vi "API String - Set Float Format String.vi"(8 "Error in":errorcluster caption="Error in (no error)", 11 "Float Format String Setting":string="%.6p") -> (0 "Error out":errorcluster, 3 "Float Format String":string)   [LabVIEW 2017, in "API String Arguments Support.lvlib"]
uses:
  API String Arguments Support.lvlib
  <userlib>/_NEVSTOP/Communicable State Machine(CSM)/Communicable State Machine.lvlib
  <userlib>/_NEVSTOP/Communicable State Machine(CSM)/_Shared/CSM Shared.lvlib
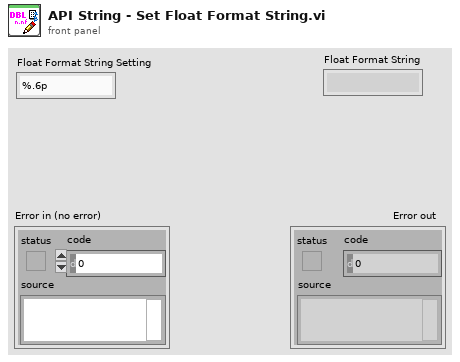
[diagram p1: front panel]
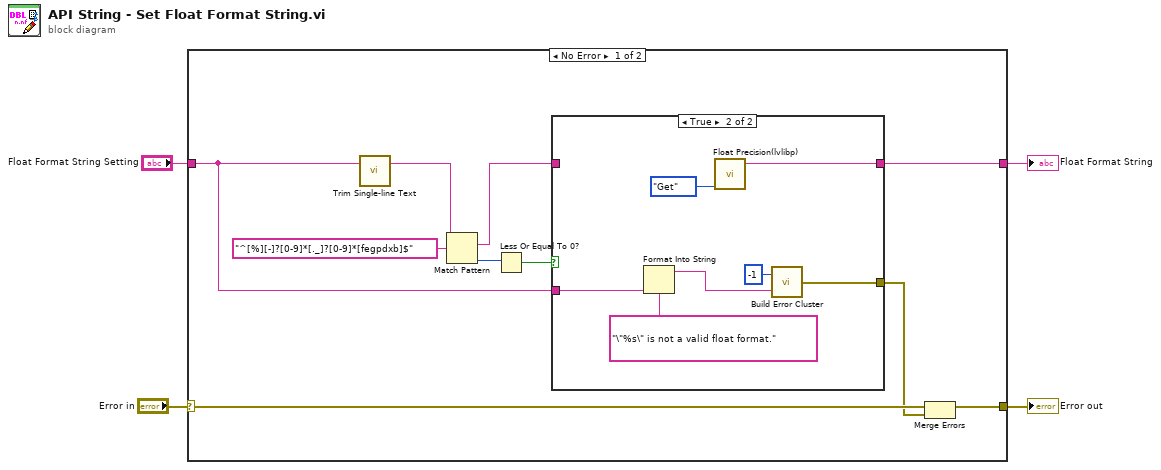
[diagram p0: block diagram]
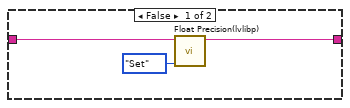
[diagram p2: hidden frame]
diagram:
  n1 = case shown="No Error" "Error in" {
    selector: "Error in" -> [w12 w25]
    tunnel: "Float Format String Setting" -> [w7 _]
    tunnel: [w11 w25] -> w2
    tunnel: [w5 _] -> w1
    frame No Error {
      n2 = call <userlib>:"Trim Single-line Text.vi"("single-line text"=w7) -> ("trimed text"=w14:string)  [unwired: 2 in]
      n3 = Match Pattern(string=w14, regular expression="^[%][-]?[0-9]*[._]?[0-9]*[fegpdxb]$") -> (match substring=w6:string, offset past match=w10:i32)  [unwired: 1 in, 2 out]
      n4 = Less Or Equal To 0?(x=w10) -> (x <= 0?=w8:bool)
      n5 = case shown="True" w8 {
        tunnel: [_ w24] -> w9
        tunnel: w7 -> [_ w22]
        tunnel: w6 -> [w16 _]
        tunnel: [w15 w18] -> w5
        frame False {
          n6 = call "Float Precision(lvlibp).vi"("Enum"=enum16{"Set", "Get"}."Set", "Precision"=w16) -> ("Format String"=w15:string)  [unwired: 9 in]
        }
        frame True {
          n7 = Format Into String(format string="\"%s\" is not a valid float format.", w22) -> (resulting string=w21:string)  [unwired: 2 in, 1 out]
          n8 = call "Float Precision(lvlibp).vi"("Enum"=enum16{"Set", "Get"}."Get") -> ("Format String"=w18:string)  [unwired: 10 in]
          n9 = call <userlib>:"Build Error Cluster.vi"("String to Prepend to Source (\"\")"=w21, "Code"=-1 ("code")) -> ("error out"=w24:errorcluster)
        }
      }
      n10 = Merge Errors(w12, w9) -> (w11:errorcluster)
    }
    frame Error {
    }
  }
  "Error out" <- w2
  "Float Format String" <- w1
